vi "sio ioctl.vi"(8 "mode":i32, 9 "baud":i32, 10 "port":i32) -> (2 "function return":i32, 3 "port":i32)   [LabVIEW 2012, in "PCOMM.lvlib"]
doc: "int WINAPI sio_ioctl(int port, int baud, int mode);"
uses:
  PCOMM.lvlib
  #001 2018-09-10/Data/PCOMM.DLL
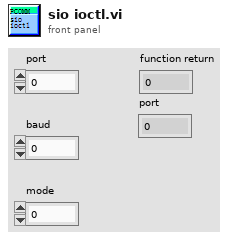
[diagram p1: front panel]
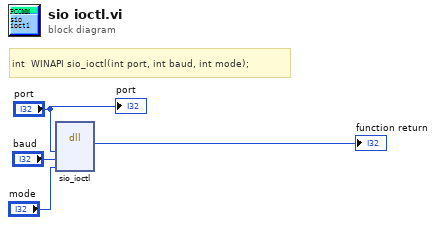
[diagram p0: block diagram]
diagram:
  # "int  WINAPI sio_ioctl(int port, int baud, int mode);"
  n1 = dll-call lib="E:/ProJect/#008 ESDMonitor/#002 Labview/#001 2018-09-10/Data/PCOMM.*" fn="sio_ioctl"("port"="port", "baud"="baud", "mode"="mode") -> (→"function return":i32)  [unwired: 6 in, 2 out]
  "port" <- "port"
